vi "clean.vi"() -> ()   [LabVIEW 2026]
panel:
  in  "Serial":refnum<visa-resource-name>
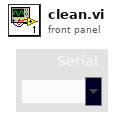
[diagram p1: front panel]
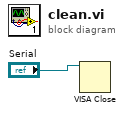
[diagram p0: block diagram]
diagram:
  n1 = VISA Close(VISA resource name="Serial") -> ()  [unwired: 1 in, 1 out]
